vi "SwerveModuleReadData.vi"(10 "NT Name (Errors)":string, 11 "NT Name (Details)":string) -> (0 "Shifter State":string, 1 "Drive Velocity":dbl format="%.1f", 2 "Drive Temperature":dbl, 3 "Azimuth Position":dbl format="%.1f", 4 "Shifter Failure":T1, 5 "Drive Overheating":T1, 6 "Drive Fault":T1, 7 "Azimuth Fault":T1)   [LabVIEW 2020]
uses:
  <vilib>/Rock Robotics/Network Tables/NT Read Numeric Array.vi
  <vilib>/Rock Robotics/Network Tables/NT Read Boolean Array.vi
  GlobalDashboard.vi
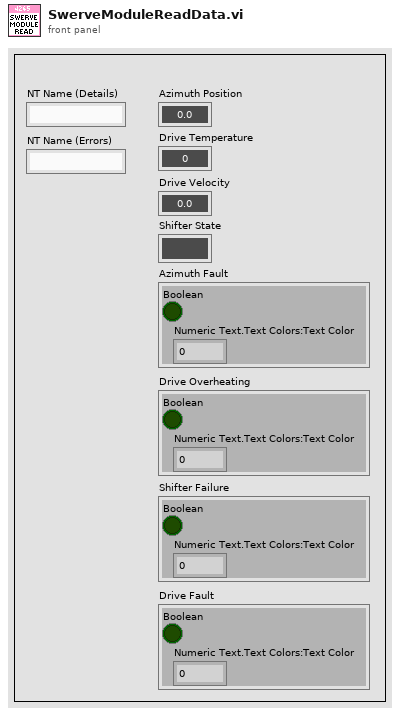
[diagram p1: front panel]
types:
  T1 = cluster{"Boolean":bool, "Numeric Text.Text Colors:Text Color":u32}
  T2 = cluster{bool, "Numeric Text.Text Colors:Text Color":u32}
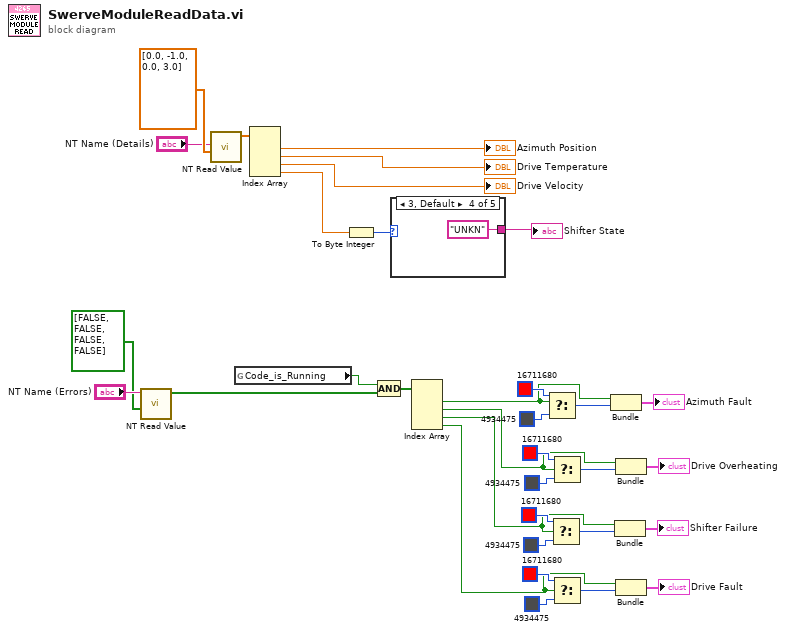
[diagram p0: block diagram]
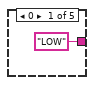
[diagram p2: hidden frame]
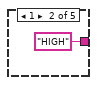
[diagram p3: hidden frame]
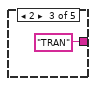
[diagram p4: hidden frame]
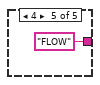
[diagram p5: hidden frame]
diagram:
  n1 = call-poly <vilib>:"NT Read Value.vi"("default value"=bool[] [FALSE, FALSE, FALSE, FALSE], "name"="NT Name (Errors)") -> ("value"=w26:bool[])  [unwired: 7 in, 2 out]
  n2 = call-poly <vilib>:"NT Read Value.vi"("default value"=dbl[] [0.0, -1.0, 0.0, 3.0] ("Default Value"), "name"="NT Name (Details)") -> ("value"=w32:dbl[])  [unwired: 7 in, 2 out]
  n3 = global read "GlobalDashboard.vi" "Code_is_Running"() -> (w8:bool)
  n4 = Index Array(array=w32) -> (element #1=→"Azimuth Position":dbl, element #2=→"Drive Temperature":dbl, element #3=→"Drive Velocity":dbl, element #4=w28:dbl)  [unwired: 4 in]
  n5 = To Byte Integer(number=w28) -> (8bit integer=w27:i8)
  n6 = Compound Arithmetic op=AND(w8, w26) -> (w9:bool[])
  n7 = case shown="3, Default" w27 {
    tunnel: ["LOW" "HIGH" "TRAN" "UNKN" "FLOW"] -> w29
    frame 0 {
    }
    frame 1 {
    }
    frame 2 {
    }
    frame 3, Default {
    }
    frame 4 {
    }
  }
  "Shifter State" <- w29
  n8 = Index Array(array=w9) -> (element #1=w22:bool, element #2=w12:bool, element #3=w2:bool, element #4=w1:bool)  [unwired: 4 in]
  n9 = Select(t=u32 16711680 ("Numeric Text.Text Colors:Text Color"), s=w22, f=u32 4934475 ("Numeric Text.Text Colors:Text Color")) -> (s? t:f=w23:u32)
  n10 = Select(t=u32 16711680 ("Numeric Text.Text Colors:Text Color"), s=w2, f=u32 4934475 ("Numeric Text.Text Colors:Text Color")) -> (s? t:f=w14:u32)
  n11 = Select(t=u32 16711680 ("Numeric Text.Text Colors:Text Color"), s=w12, f=u32 4934475 ("Numeric Text.Text Colors:Text Color")) -> (s? t:f=w18:u32)
  n12 = Select(t=u32 16711680 ("Numeric Text.Text Colors:Text Color"), s=w1, f=u32 4934475 ("Numeric Text.Text Colors:Text Color")) -> (s? t:f=w4:u32)
  n13 = Bundle(w22, "Numeric Text.Text Colors:Text Color"=w23) -> (→"Azimuth Fault":T2)  [unwired: 1 in]
  n14 = Bundle(w2, "Numeric Text.Text Colors:Text Color"=w14) -> (→"Shifter Failure":T2)  [unwired: 1 in]
  n15 = Bundle(w12, "Numeric Text.Text Colors:Text Color"=w18) -> (→"Drive Overheating":T2)  [unwired: 1 in]
  n16 = Bundle(w1, "Numeric Text.Text Colors:Text Color"=w4) -> (→"Drive Fault":T2)  [unwired: 1 in]
